vi "EnglishTeacher.vi"() -> ()   [LabVIEW 2020]
uses:
  #typedef_States.ctl
  #typedef_CurrentMode.ctl
  #typedef_Database.ctl
  #typedef_Word.ctl
  #typedef_TimerAction.ctl
panel:
  in  "Angielski":string
  in  "Exit":bool caption="E"
  in  "Stop":bool caption="S"
  in  "Start Test":bool
  in  "Start Learning":bool
  out "Angielski":string
  out "Polski":string
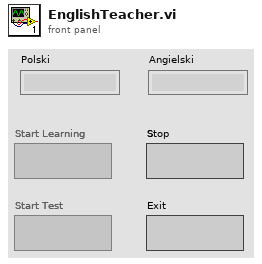
[diagram p1: front panel]
types:
  T1 = typedef "#typedef_States.ctl" = enum16{"Initialize", "Idle", "Select Mode", "L_ShowPL", "Wait3sec", "L_ShowENG", "L_Empty", "T_ShowPL", "Wait5sec", "T_WriteENG", "T_Check", "T_Wait", "Stop", "End"}
  T2 = typedef "#typedef_Word.ctl" = cluster{"Polski":string, "Angielski":string}
  T3 = typedef "#typedef_Database.ctl" = cluster{"Current Mode":T4, "Word's Database":T2[], "Word":T2, "Current Word Index":i32, "Previous State":T1}
  T4 = typedef "#typedef_CurrentMode.ctl" = u16
  T5 = typedef "#typedef_TimerAction.ctl" = enum16{"Reset", "TimeElapsed"}
  T6 = enum8{"Enabled", "Disabled", "Disabled and Grayed Out"}
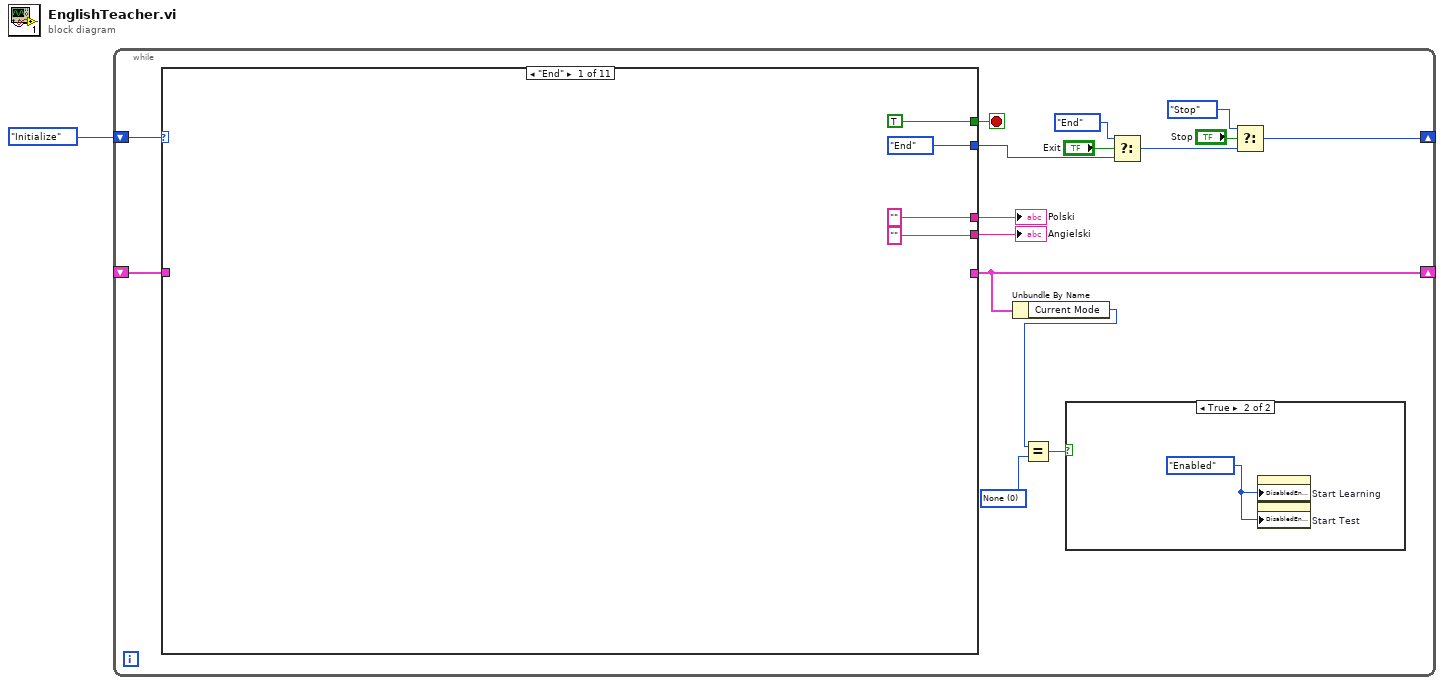
[diagram p0: block diagram]
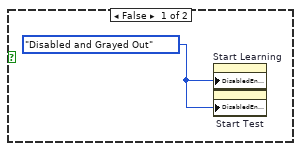
[diagram p2: hidden frame]
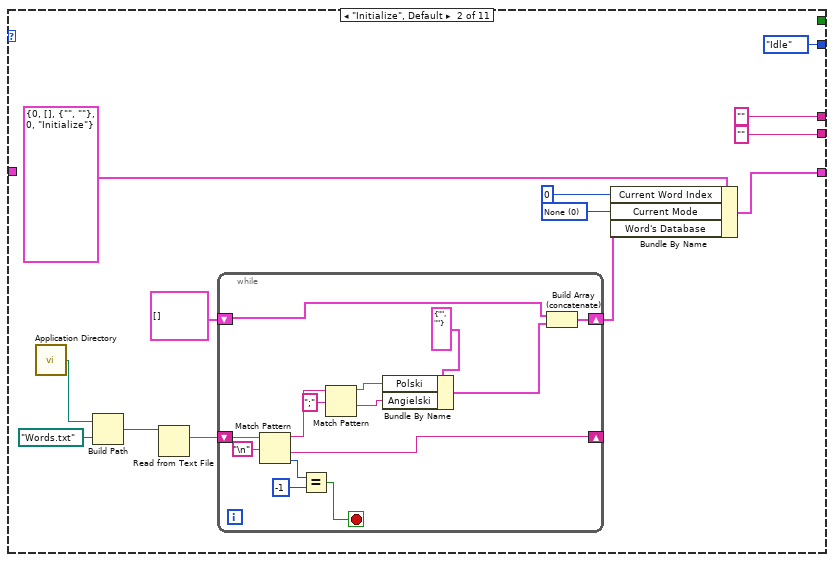
[diagram p3: hidden frame]
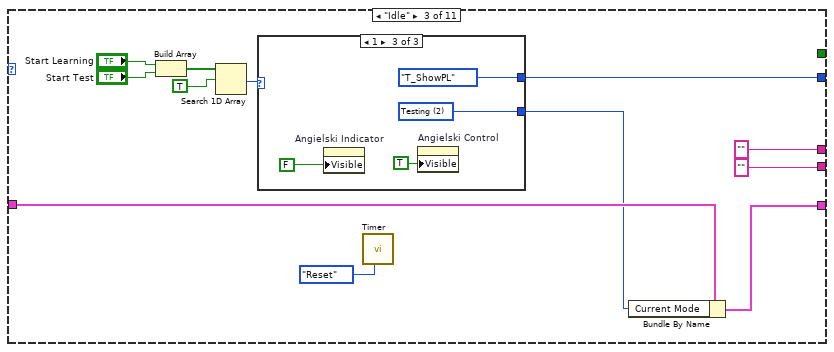
[diagram p4: hidden frame]
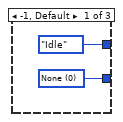
[diagram p5: hidden frame]
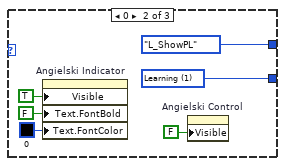
[diagram p6: hidden frame]
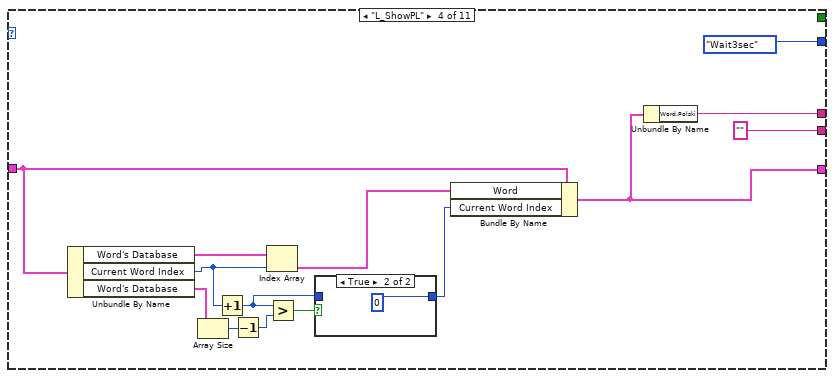
[diagram p7: hidden frame]
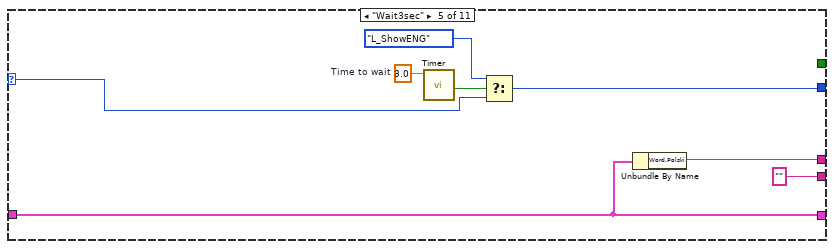
[diagram p9: hidden frame]
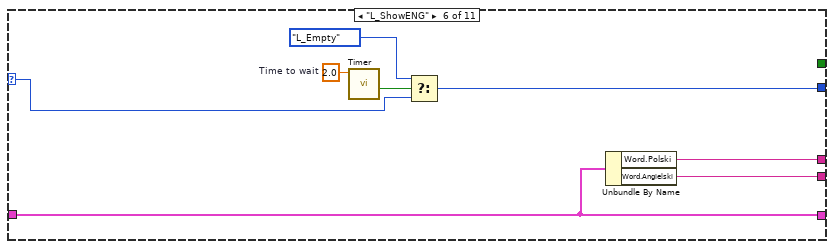
[diagram p10: hidden frame]
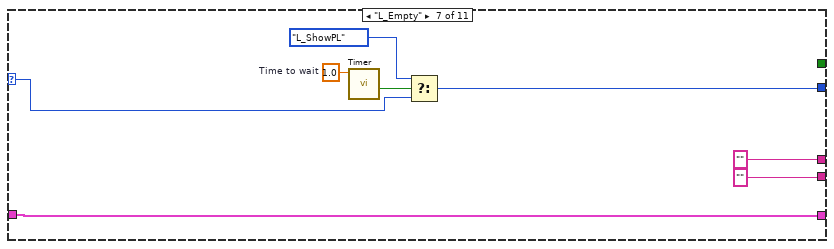
[diagram p11: hidden frame]
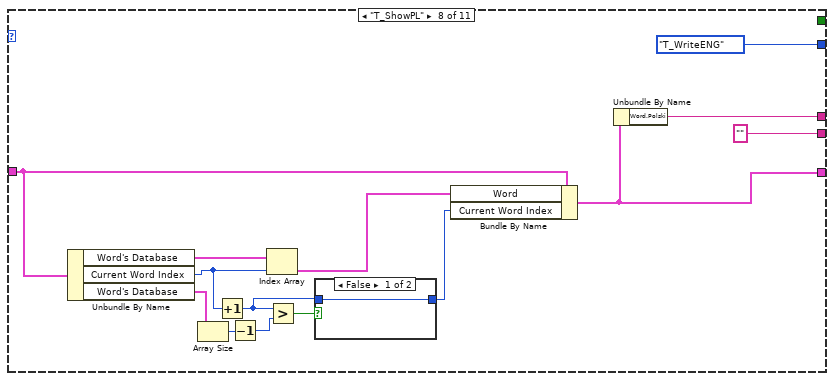
[diagram p12: hidden frame]
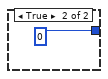
[diagram p13: hidden frame]
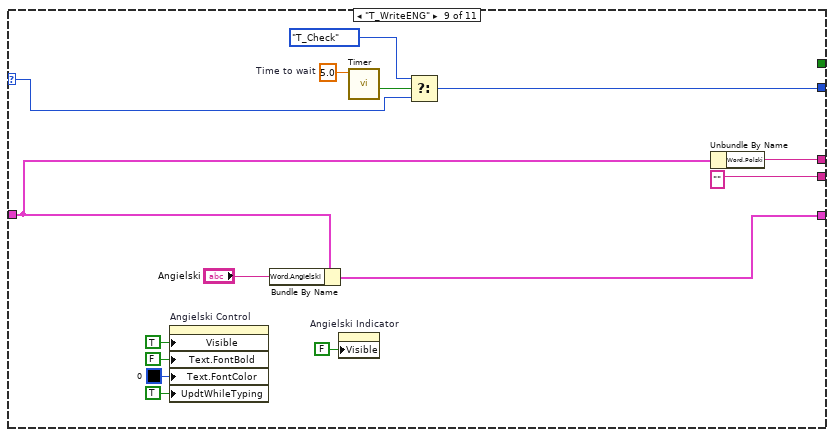
[diagram p14: hidden frame]
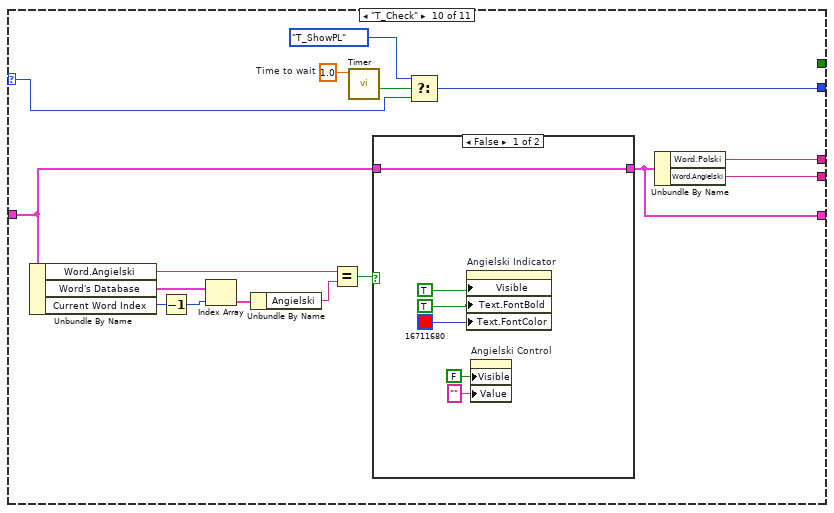
[diagram p15: hidden frame]
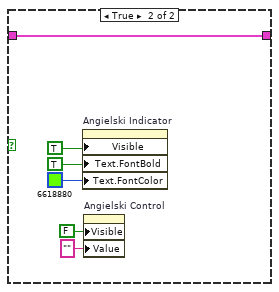
[diagram p16: hidden frame]
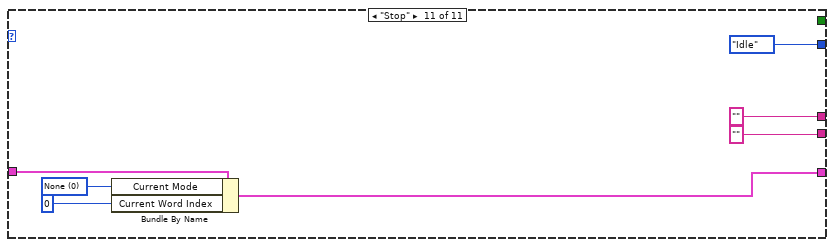
[diagram p17: hidden frame]
diagram:
  n1 = while {
    shift-right: [w9] -> _
    shift-left: #typedef_States."Initialize" ("States") -> [w17]
    shift-right: [w5] -> _
    shift-left: _ -> [w8]
    stop <- w16 stop-if-true
    w3 = T4 0 items=["None", "Learning", "Testing"] ("y")
    n2 = case shown="\"End\"" w17 {
      selector: w17 -> [_ _ _ _ w94 w103 w112 _ w143 w159 _]
      tunnel: [_ w32 w56 w80 w93 w100 w109 w119 w136 w147 w176] -> w5
      tunnel: [#typedef_States."End" ("States") #typedef_States."Idle" ("States") w55 #typedef_States."Wait3sec" ("States") w95 w101 w110 #typedef_States."T_WriteENG" ("States") w141 w157 #typedef_States."Idle" ("States")] -> w13
      tunnel: [TRUE _ _ _ _ _ _ _ _ _ _] -> w16
      tunnel: w8 -> [_ _ w57 w88 w93 w100 w109 w127 w138 w148 w179]
      tunnel: ["" ("Polski") "" ("Polski") "" ("Polski") w79 w92 w106 "" ("Polski") w118 w140 w156 "" ("Polski")] -> w7
      tunnel: ["" ("Angielski") "" ("Angielski") "" ("Angielski") "" ("Angielski") "" ("Angielski") w99 "" ("Angielski") "" ("Angielski") "" ("Angielski") w149 "" ("Angielski")] -> w6
      frame "End" {
      }
      frame "Initialize", Default {
        w24 = T4 0 items=["None", "Learning", "Testing"] ("Current Mode")
        n3 = call <vilib>:"Application Directory.vi"() -> ("Application Directory"=w36:path)
        n4 = Build Path(base path=w36, name or relative path=path "Words.txt") -> (appended path=w34:path)
        n5 = Read from Text File(file (use dialog)=w34) -> (text=w27:string)  [unwired: 3 in, 3 out]
        n6 = while {
          shift-right: [w46] -> _
          shift-left: w27 -> [w50]
          shift-right: [w40] -> w31
          shift-left: T2[] [] -> [w39]
          stop <- w38 stop-if-true
          n7 = Match Pattern(string=w50, regular expression="\n") -> (before substring=w45:string, after substring=w46:string, offset past match=w48:i32)  [unwired: 1 in, 1 out]
          n8 = Equal?(x=w48, y=-1) -> (x = y?=w38:bool)
          n9 = Match Pattern(string=w45, regular expression=";") -> (before substring=w43:string, after substring=w42:string)  [unwired: 1 in, 2 out]
          n10 = Bundle By Name(cluster=T2 {"Polski"="", "Angielski"=""} ("Word"), "Polski"=w43, "Angielski"=w42) -> (w41:T2)
          n11 = Build Array (concatenate)(w39, w41) -> (w40:T2[])
        }
        n12 = Bundle By Name(cluster=T3 {"Current Mode"=0, "Word's Database"=[], "Word"={"Polski"="", "Angielski"=""}, "Current Word Index"=0, "Previous State"=enum."Initialize"} ("Database"), "Current Word Index"=0, "Current Mode"=w24, "Word's Database"=w31) -> (w32:T3)
      }
      frame "Idle" {
        n13 = Build Array("Start Learning", "Start Test") -> (w60:bool[])
        n14 = Search 1D Array(1D array=w60, element=TRUE) -> (index of element=w58:i32)  [unwired: 1 in]
        n15 = case shown="1" w58 {
          tunnel: [#typedef_States."Idle" ("States") #typedef_States."L_ShowPL" ("States") #typedef_States."T_ShowPL" ("States")] -> w55
          tunnel: [w64 w69 w73] -> w54
          frame -1, Default {
            w64 = T4 0 items=["None", "Learning", "Testing"] ("Current Mode")
          }
          frame 0 {
            w69 = T4 1 items=["None", "Learning", "Testing"] ("Current Mode")
            n16 = property on="Angielski Indicator" class="Str"("Visible"=TRUE, "Text.FontBold"=FALSE ("Text.Font:Bold"), "Text.FontColor"=u32 0 ("Text.Font:Color")) -> ()  [unwired: 2 in, 2 out]
            n17 = property on="Angielski Control" class="Str"("Visible"=FALSE) -> ()  [unwired: 2 in, 2 out]
          }
          frame 1 {
            w73 = T4 2 items=["None", "Learning", "Testing"] ("Current Mode")
            n18 = property on="Angielski Indicator" class="Str"("Visible"=FALSE) -> ()  [unwired: 2 in, 2 out]
            n19 = property on="Angielski Control" class="Str"("Visible"=TRUE) -> ()  [unwired: 2 in, 2 out]
          }
        }
        n20 = call "Timer.vi"("Action"=#typedef_TimerAction."Reset") -> ()  [unwired: 9 in, 2 out]
        n21 = Bundle By Name(cluster=w57, "Current Mode"=w54) -> (w56:T3)
      }
      frame "L_ShowPL" {
        n22 = Unbundle By Name(w88) -> ("Word's Database"=w77:T2[], "Current Word Index"=w84:i32, "Word's Database"=w86:T2[])
        n23 = Array Size(array=w86) -> (size(s)=w85:i32)
        n24 = Increment(x=w84) -> (x+1=w81:i32)
        n25 = Decrement(x=w85) -> (x-1=w75:i32)
        n26 = Index Array(array=w77, index=w84) -> (element=w87:T2)
        n27 = Greater?(x=w81, y=w75) -> (0:w83:bool)
        n28 = case shown="True" w83 {
          tunnel: [w89 0] -> w82
          tunnel: w81 -> [w89 _]
          frame False {
          }
          frame True {
          }
        }
        n29 = Bundle By Name(cluster=w88, "Word"=w87, "Current Word Index"=w82) -> (w80:T3)
        n30 = Unbundle By Name(w80) -> ("Word.Polski"=w79:string)
      }
      frame "Wait3sec" {
        w98 = 3.0  # Time to wait
        n31 = call "Timer.vi"("Limit"=w98) -> ("Over limit?"=w97:bool)  [unwired: 9 in, 1 out]
        n32 = Select(t=#typedef_States."L_ShowENG" ("States"), s=w97, f=w94) -> (s? t:f=w95:T1)
        n33 = Unbundle By Name(w93) -> ("Word.Polski"=w92:string)
      }
      frame "L_ShowENG" {
        w105 = 2.0  # Time to wait
        n34 = call "Timer.vi"("Limit"=w105) -> ("Over limit?"=w104:bool)  [unwired: 9 in, 1 out]
        n35 = Select(t=#typedef_States."L_Empty" ("States"), s=w104, f=w103) -> (s? t:f=w101:T1)
        n36 = Unbundle By Name(w100) -> ("Word.Polski"=w106:string, "Word.Angielski"=w99:string)
      }
      frame "L_Empty" {
        w114 = 1.0  # Time to wait
        n37 = call "Timer.vi"("Limit"=w114) -> ("Over limit?"=w113:bool)  [unwired: 9 in, 1 out]
        n38 = Select(t=#typedef_States."L_ShowPL" ("States"), s=w113, f=w112) -> (s? t:f=w110:T1)
      }
      frame "T_ShowPL" {
        n39 = Unbundle By Name(w127) -> ("Word's Database"=w128:T2[], "Current Word Index"=w123:i32, "Word's Database"=w125:T2[])
        n40 = Array Size(array=w125) -> (size(s)=w124:i32)
        n41 = Increment(x=w123) -> (x+1=w120:i32)
        n42 = Decrement(x=w124) -> (x-1=w115:i32)
        n43 = Index Array(array=w128, index=w123) -> (element=w126:T2)
        n44 = Greater?(x=w120, y=w115) -> (0:w122:bool)
        n45 = case shown="False" w122 {
          tunnel: [w129 0] -> w121
          tunnel: w120 -> [w129 _]
          frame False {
          }
          frame True {
          }
        }
        n46 = Bundle By Name(cluster=w127, "Word"=w126, "Current Word Index"=w121) -> (w119:T3)
        n47 = Unbundle By Name(w119) -> ("Word.Polski"=w118:string)
      }
      frame "T_WriteENG" {
        w145 = 5.0  # Time to wait
        n48 = property on="Angielski Control" class="Str"("Visible"=TRUE ("Update While Typing?"), "Text.FontBold"=FALSE ("Text.Font:Bold"), "Text.FontColor"=u32 0 ("Text.Font:Color"), "UpdtWhileTyping"=TRUE ("Update While Typing?")) -> ()  [unwired: 2 in, 2 out]
        n49 = Bundle By Name(cluster=w138, "Word.Angielski"="Angielski") -> (w136:T3)
        n50 = property on="Angielski Indicator" class="Str"("Visible"=FALSE) -> ()  [unwired: 2 in, 2 out]
        n51 = call "Timer.vi"("Limit"=w145) -> ("Over limit?"=w144:bool)  [unwired: 9 in, 1 out]
        n52 = Select(t=#typedef_States."T_Check" ("States"), s=w144, f=w143) -> (s? t:f=w141:T1)
        n53 = Unbundle By Name(w138) -> ("Word.Polski"=w140:string)
      }
      frame "T_Check" {
        w161 = 1.0  # Time to wait
        n54 = Unbundle By Name(w148) -> ("Word.Angielski"=w152:string, "Word's Database"=w155:T2[], "Current Word Index"=w154:i32)
        n55 = Decrement(x=w154) -> (x-1=w146:i32)
        n56 = Index Array(array=w155, index=w146) -> (element=w153:T2)
        n57 = Unbundle By Name(w153) -> ("Angielski"=w151:string)
        n58 = Equal?(x=w152, y=w151) -> (x = y?=w150:bool)
        n59 = call "Timer.vi"("Limit"=w161) -> ("Over limit?"=w160:bool)  [unwired: 9 in, 1 out]
        n60 = case shown="False" w150 {
          tunnel: w148 -> [w162 w168]
          tunnel: [w162 w168] -> w147
          frame False {
            n61 = property on="Angielski Indicator" class="Str"("Visible"=TRUE, "Text.FontBold"=TRUE ("Text.Font:Bold"), "Text.FontColor"=u32 16711680 ("Text.Font:Color")) -> ()  [unwired: 2 in, 2 out]
            n62 = property on="Angielski Control" class="Str"("Visible"=FALSE, "Value"="" ("Angielski")) -> ()  [unwired: 2 in, 2 out]
          }
          frame True {
            n63 = property on="Angielski Indicator" class="Str"("Visible"=TRUE, "Text.FontBold"=TRUE ("Text.Font:Bold"), "Text.FontColor"=u32 6618880 ("Text.Font:Color")) -> ()  [unwired: 2 in, 2 out]
            n64 = property on="Angielski Control" class="Str"("Visible"=FALSE, "Value"="" ("Angielski")) -> ()  [unwired: 2 in, 2 out]
          }
        }
        n65 = Select(t=#typedef_States."T_ShowPL" ("States"), s=w160, f=w159) -> (s? t:f=w157:T1)
        n66 = Unbundle By Name(w147) -> ("Word.Polski"=w156:string, "Word.Angielski"=w149:string)
      }
      frame "Stop" {
        w178 = T4 0 items=["None", "Learning", "Testing"] ("Current Mode")
        n67 = Bundle By Name(cluster=w179, "Current Mode"=w178, "Current Word Index"=0) -> (w176:T3)
      }
    }
    "Polski" <- w7
    "Angielski" <- w6
    n68 = Unbundle By Name(w5) -> ("Current Mode"=w4:T4)
    n69 = Equal?(x=w4, y=w3) -> (x = y?=w2:bool)
    n70 = case shown="True" w2 {
      frame False {
        w18 = T6."Disabled and Grayed Out" ("Disabled")
        n71 = property on="Start Learning" class="Bool"("DisabledEnum"=w18) -> ()  [unwired: 2 in, 2 out]
        n72 = property on="Start Test" class="Bool"("DisabledEnum"=w18) -> ()  [unwired: 2 in, 2 out]
      }
      frame True {
        w19 = T6."Enabled" ("Disabled")
        n73 = property on="Start Learning" class="Bool"("DisabledEnum"=w19) -> ()  [unwired: 2 in, 2 out]
        n74 = property on="Start Test" class="Bool"("DisabledEnum"=w19) -> ()  [unwired: 2 in, 2 out]
      }
    }
    n75 = Select(t=#typedef_States."End" ("States"), s="Exit", f=w13) -> (s? t:f=w12:T1)
    n76 = Select(t=#typedef_States."Stop" ("States"), s="Stop", f=w12) -> (s? t:f=w9:T1)
  }
